vi "Post-Build Action.vi"(5 "Files Generated by Build":path[](array[path]), 6 "Top Level/Always Included VIs":path[](array[path]), 7 "Destination Path":path, 8 "error in (no error)":errorcluster, 9 "Target Name":string, 10 "Build Specification Name":string, 11 "Project Path":path) -> (0 "error out":errorcluster)   [LabVIEW 2014]
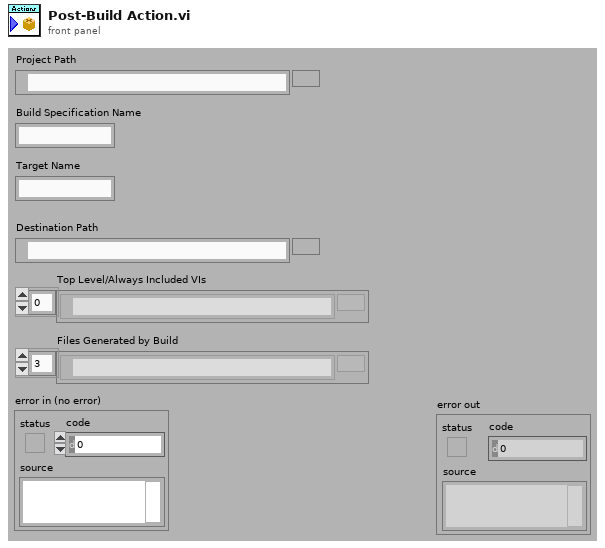
[diagram p1: front panel]
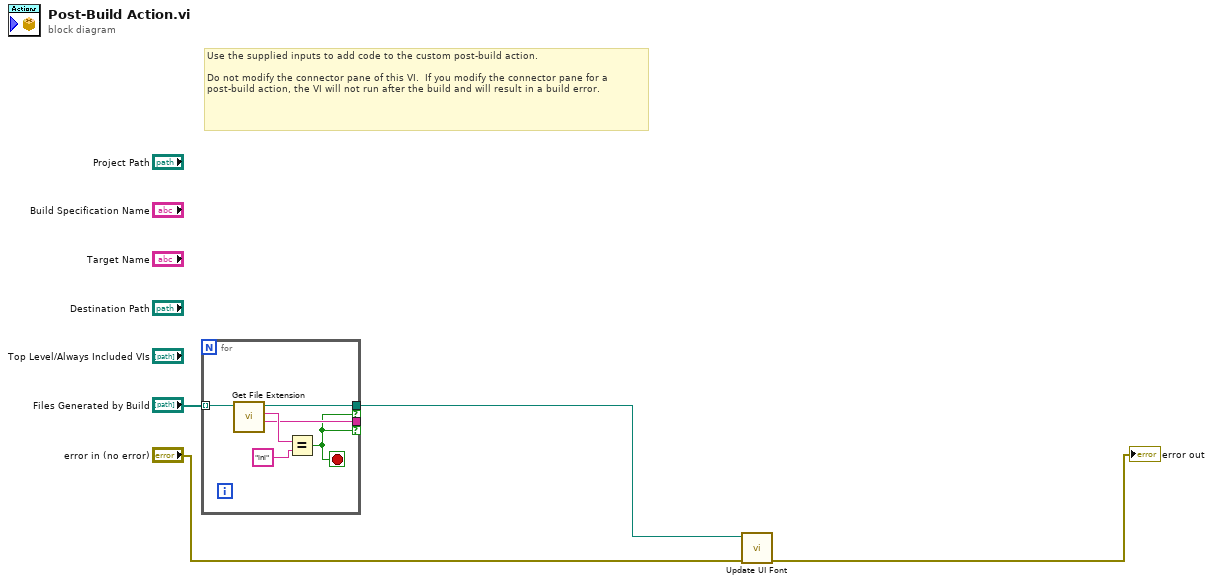
[diagram p0: block diagram]
diagram:
  # "Use the supplied inputs to add code to the custom post-build action.\n\nDo not modify the connector pane of this VI.  If you modify the connector pane for a post-build action, the VI will not run after the build and will result in a build error."
  n1 = for {
    tunnel: "Files Generated by Build" -> [w10] mode=indexing
    tunnel: [w9] -> w1 if=w5
    tunnel: [w6] -> _ if=w5
    stop <- w5 stop-if-true
    n2 = call <vilib>:"Get File Extension.vi"("file"=w10) -> ("filename without extension"=w6:string, "lowercase file extension"=w8:string, "dup file"=w9:path)  [unwired: 7 in, 1 out]
    n3 = Equal?(x=w8, y="ini" ("string")) -> (x = y?=w5:bool)
  }
  n4 = call "Update UI Font.vi"("error in (no error)"="error in (no error)", "dup file"=w1) -> ("error out"=→"error out":errorcluster)  [unwired: 8 in, 1 out]
